vi "XmlRpcServerRequestEventCallback.vi"(4 "User Parameter":T1, 5 "Event Data":T2, 6 "Control Ref":refnum<k24>, 7 "Event Common Data":T3) -> ()   [LabVIEW 2014]
uses:
  Z:/Samples/Libraries/net35/UnderAutomation.UniversalRobots.dll
  Libraries/net35/UnderAutomation.UniversalRobots.dll
panel:
  # "This VI is called when a XML RPC request is sent from the robot to the LabView program"
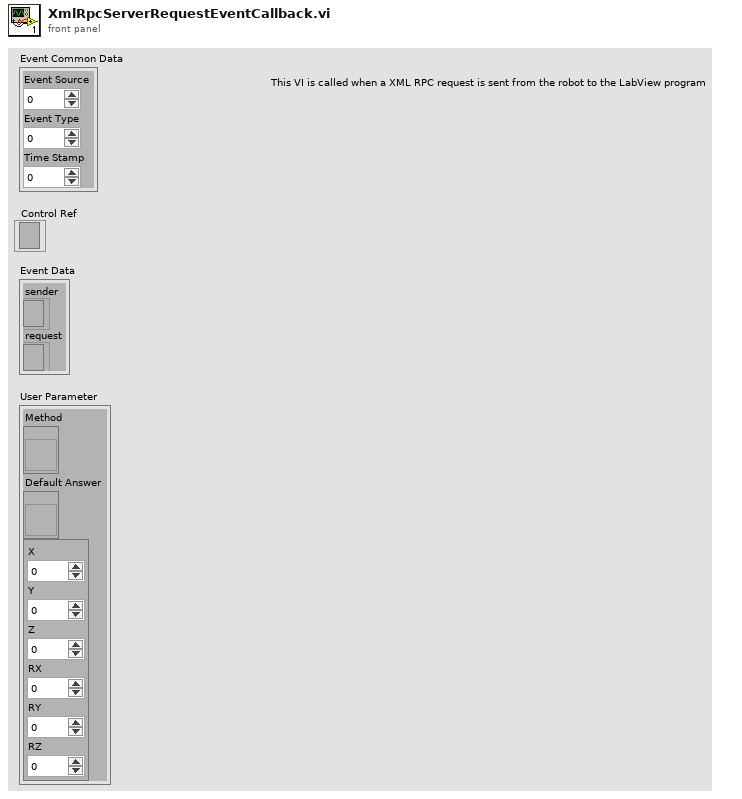
[diagram p1: front panel]
types:
  T1 = cluster{"Method":refnum<vi>, "Default Answer":refnum<vi>, cluster{"X":dbl, "Y":dbl, "Z":dbl, "RX":dbl, "RY":dbl, "RZ":dbl}}
  T2 = cluster{"sender":refnum<k24>, "request":refnum<k24>}
  T3 = cluster{"Event Source":i32, "Event Type":u32, "Time Stamp":u32}
  T4 = cluster{"X":dbl, "Y":dbl, "Z":dbl, "RX":dbl, "RY":dbl, "RZ":dbl}
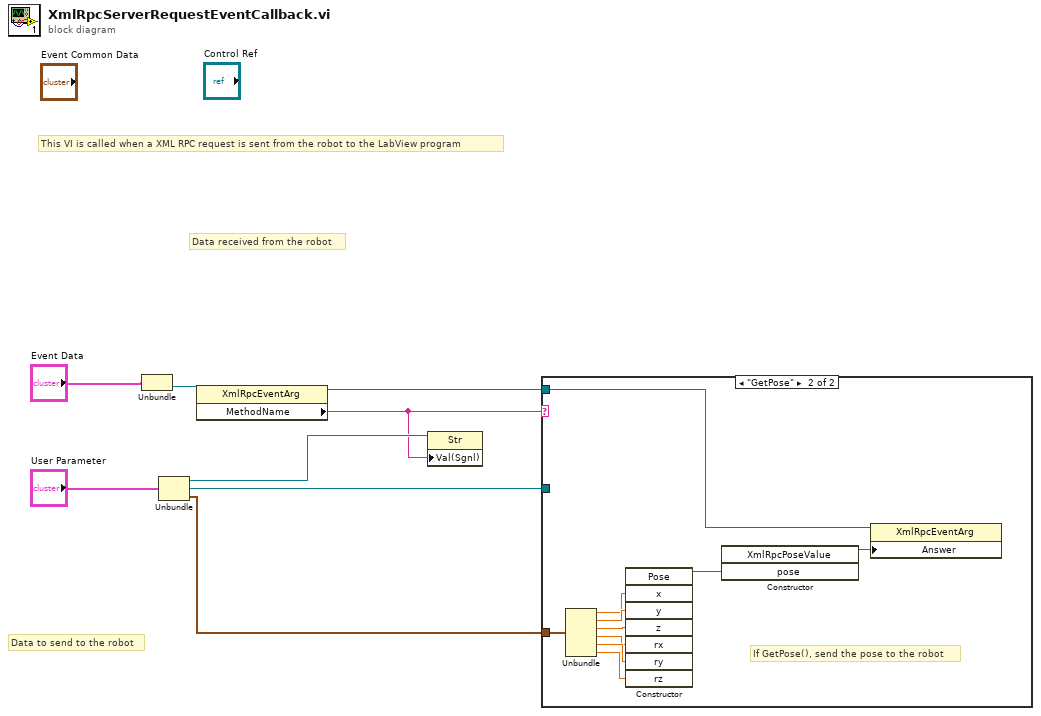
[diagram p0: block diagram]
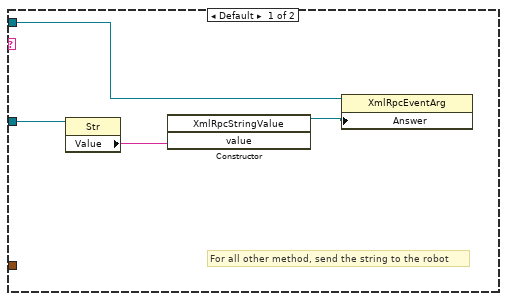
[diagram p2: hidden frame]
diagram:
  # "This VI is called when a XML RPC request is sent from the robot to the LabView program"
  # "Data to send to the robot"
  # "Data received from the robot"
  n1 = Unbundle("Event Data") -> ("request"=w6:refnum<k24>)  [unwired: 1 out]
  n2 = Unbundle("User Parameter") -> ("Method"=w5:refnum<vi>, "Default Answer"=w2:refnum<vi>, w3:T4)
  n3 = property class="XmlRpcEventArg"(reference=w6) -> (reference out=w1:refnum<k24>, "MethodName"=w4:string)  [unwired: 1 in, 1 out]
  n4 = property class="Str"(reference=w5, "Val(Sgnl)"=w4) -> ()  [unwired: 1 in, 2 out]
  n5 = case shown="\"GetPose\"" w4 {
    tunnel: w3 -> [_ w16]
    tunnel: w2 -> [w12 _]
    tunnel: w1 -> [w10 w14]
    frame Default {
      # "For all other method, send the string to the robot"
      n6 = property class="Str"(reference=w12) -> ("Value"=w11:string)  [unwired: 1 in, 2 out]
      n7 = constructor class="XmlRpcStringValue"("value"=w11) -> (reference out=w9:refnum<k24>)  [unwired: 3 in, 3 out]
      n8 = property class="XmlRpcEventArg"(reference=w10, "Answer"=w9) -> ()  [unwired: 1 in, 2 out]
    }
    frame "GetPose" {
      # "If GetPose(), send the pose to the robot"
      n9 = Unbundle(w16) -> ("X"=w17:dbl, "Y"=w18:dbl, "Z"=w19:dbl, "RX"=w20:dbl, "RY"=w21:dbl, "RZ"=w22:dbl)
      n10 = constructor class="Pose"("x"=w17, "y"=w18, "z"=w19, "rx"=w20, "ry"=w21, "rz"=w22) -> (reference out=w15:refnum<k24>)  [unwired: 3 in, 8 out]
      n11 = constructor class="XmlRpcPoseValue"("pose"=w15) -> (reference out=w13:refnum<k24>)  [unwired: 3 in, 3 out]
      n12 = property class="XmlRpcEventArg"(reference=w14, "Answer"=w13) -> ()  [unwired: 1 in, 2 out]
    }
  }
